vi "testing_delay_sweep.vi"() -> ()   [LabVIEW 2015, in "Tausand AB1000.lvlib"]
uses:
  <instrlib>/Tausand AB1000/Tausand AB1000.lvlib
  <instrlib>/Tausand AB1000/Public/Controls/deviceTypeRing.ctl
  <instrlib>/Tausand AB1000/Public/Controls/counters4ch.ctl
  <instrlib>/Tausand AB1000/Public/Controls/channelRing.ctl
panel:
  in  "delayed channel":T1=1 items=["none", "A", "B", "C", "D", "E", "F", "G", "H"]
  in  "cw (ns)":u32=10
  out "i case":i32
  out "total cases":i32
  in  "Stop Button":bool
  out "coinc Chart":T2(graph)
  out "current values":T3
  in  "sampling (ms)":u32=1000
  out "i delay":i32
  out "device type":T4 items=["any"=0, "AB1002"=1002, "AB1004"=1004, "AB1502"=1502, "AB1504"=1504, "AB1902"=1902, "AB1904"=1904]
  out "delay array":u32[](array[numeric])
  in  "step delay":u32=1
  in  "max delay":u32=20
  in  "min delay":u32
  out "current delay (ns)":u32
  in  "VISA resource name":refnum<visa-resource-name>
  # "case"
  # "out of"
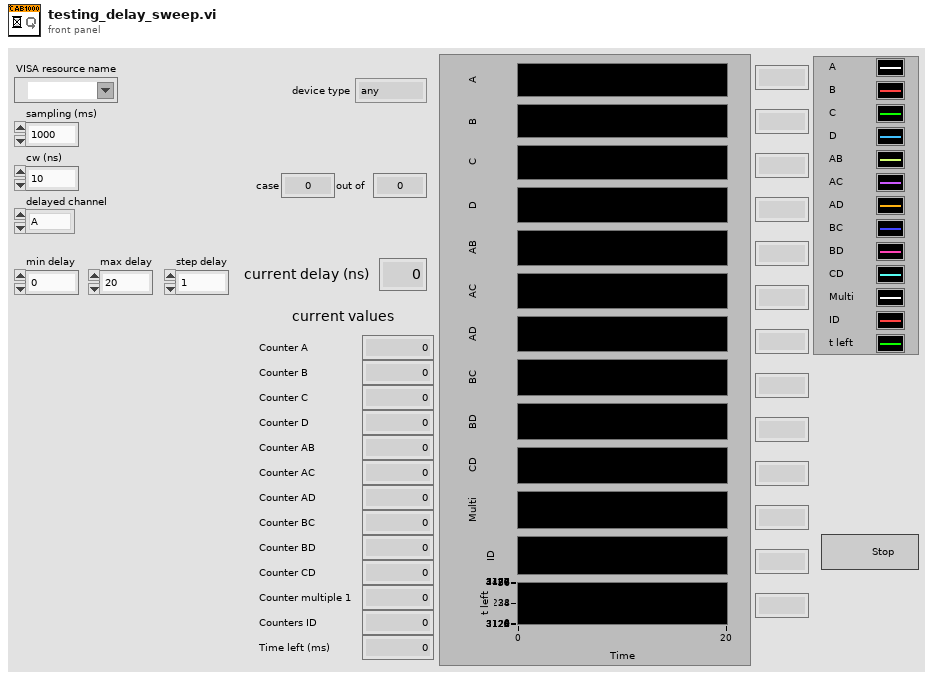
[diagram p1: front panel]
types:
  T1 = typedef "Tausand AB1000.lvlib/channelRing.ctl" = u8
  T2 = cluster{"counter_A":u32, "counter_B":u32, "counter_C":u32, "counter_D":u32, "counter_AB":u32, "counter_AC":u32, "counter_AD":u32, "counter_BC":u32, "counter_BD":u32, "counter_CD":u32, "counter_multiple_1":u32, "counters_ID":u32, "time_left":u32}
  T3 = typedef "Tausand AB1000.lvlib/counters4ch.ctl" = cluster{"counter_A":u32, "counter_B":u32, "counter_C":u32, "counter_D":u32, "counter_AB":u32, "counter_AC":u32, "counter_AD":u32, "counter_BC":u32, "counter_BD":u32, "counter_CD":u32, "counter_multiple_1":u32, "counters_ID":u32, "time_left":u32}
  T4 = typedef "Tausand AB1000.lvlib/deviceTypeRing.ctl" = u16
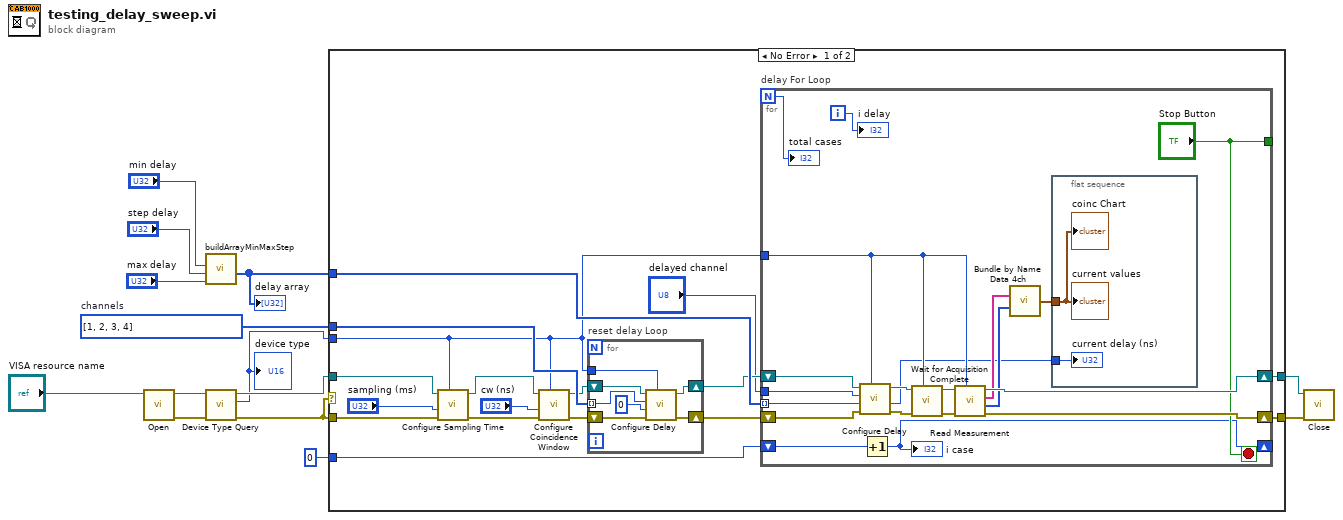
[diagram p0: block diagram]
diagram:
  w5 = T1[] [1, 2, 3, 4] items=["none", "A", "B", "C", "D", "E", "F", "G", "H"]  # channels
  n1 = call <instrlib>:"Open.vi"("VISA resource name"="VISA resource name") -> ("error out"=w10:errorcluster, "VISA resource name out"=w9:refnum<visa-resource-name>)  [unwired: 9 in]
  n2 = call <instrlib>:"buildArrayMinMaxStep.vi"("max (10)"="max delay", "step (1)"="step delay", "min (0)"="min delay") -> ("array"=w6:i32[])  [unwired: 8 in]
  "delay array" <- w6
  n3 = call <instrlib>:"Device Type Query.vi"("error in (no error)"=w10, "VISA Refnum in"=w9) -> ("error out"=w2:errorcluster, "device type"=w7:T4, "VISA Refnum out"=w8:refnum<visa-resource-name>)  [unwired: 7 in]
  "device type" <- w7
  n4 = case shown="No Error" w2 {
    tunnel: w2 -> [w26 w62]
    tunnel: w8 -> [w27 w61]
    tunnel: w7 -> [w25 _]
    tunnel: w6 -> [w31 _]
    tunnel: w5 -> [w28 _]
    tunnel: [w30 w61] -> w4
    tunnel: [w29 w62] -> w3
    tunnel: 0 ("i delay") -> [w21 _]
    frame No Error {
      n5 = call <instrlib>:"Configure Sampling Time.vi"("device type"=w25, "error in (no error)"=w26, "value (1000 ms)"="sampling (ms)", "VISA Refnum in"=w27) -> ("error out"=w23:errorcluster, "VISA Refnum out"=w22:refnum<visa-resource-name>)  [unwired: 5 in, 1 out]
      n6 = call <instrlib>:"Configure Coincidence Window.vi"("device type"=w25, "error in (no error)"=w23, "value ns (10ns)"="cw (ns)", "VISA Refnum in"=w22) -> ("error out"=w19:errorcluster, "VISA Refnum out"=w20:refnum<visa-resource-name>)  [unwired: 5 in, 1 out]
      n7 = for "reset delay Loop" {
        tunnel: w28 -> [w37] mode=indexing
        tunnel: w25 -> [w35]
        shift-right: [w33] -> w16
        shift-left: w19 -> [w34]
        shift-right: [w32] -> w17
        shift-left: w20 -> [w38]
        n8 = call <instrlib>:"Configure Delay.vi"("device type"=w35, "error in (no error)"=w34, "value (0 ns)"=u32 0, "channel"=w37, "VISA Refnum in"=w38) -> ("error out"=w33:errorcluster, "VISA Refnum out"=w32:refnum<visa-resource-name>)  [unwired: 4 in, 1 out]
      }
      n9 = for "delay For Loop" {
        N -> [w40]
        tunnel: w31 -> [w58] mode=indexing
        tunnel: w25 -> [w49]
        shift-right: [w55] -> w29
        shift-left: w16 -> [w56]
        shift-right: [w54] -> w30
        shift-left: w17 -> [w57]
        tunnel: ["Stop Button"] -> _
        shift-right: [w42] -> _
        shift-left: w21 -> [w43]
        tunnel: "delayed channel" -> [w41]
        i -> [w44]
        stop <- "Stop Button" stop-if-true
        n10 = call <instrlib>:"Configure Delay.vi"("device type"=w49, "error in (no error)"=w56, "value (0 ns)"=w58, "channel"=w41, "VISA Refnum in"=w57) -> ("error out"=w53:errorcluster, "value ns out"=w39:u32, "VISA Refnum out"=w51:refnum<visa-resource-name>)  [unwired: 4 in]
        n11 = Increment(x=w43) -> (x+1=w42:i32)
        "i case" <- w42
        n12 = call <instrlib>:"Wait for Acquisition Complete.vi"("device type"=w49, "error in (no error)"=w53, "VISA resource name"=w51) -> ("error out"=w52:errorcluster, "VISA resource name out"=w50:refnum<visa-resource-name>)  [unwired: 7 in]
        n13 = call <instrlib>:"Read Measurement.vi"("device type"=w49, "error in (no error)"=w52, "VISA Refnum in"=w50) -> ("error out"=w55:errorcluster, "values"=w47:u32[], "labels"=w48:string[], "VISA Refnum out"=w54:refnum<visa-resource-name>)  [unwired: 3 in, 2 out]
        n14 = call <instrlib>:"Bundle by Name Data 4ch.vi"("names"=w48, "values"=w47) -> ("output cluster 4ch"=w46:T3)  [unwired: 13 in]
        n15 = flat-sequence {
          tunnel: w46 -> [w60]
          tunnel: w39 -> [w59]
          frame #0 {
            "current values" <- w60
            "coinc Chart" <- w60
            "current delay (ns)" <- w59
          }
        }
        "i delay" <- w44
        "total cases" <- w40
      }
    }
    frame Error {
    }
  }
  n16 = call <instrlib>:"Close.vi"("error in (no error)"=w3, "VISA resource name"=w4) -> ()  [unwired: 9 in, 1 out]
